vi "读取检测值.vi"(8 "error in (no error)":errorcluster caption="错误输入（无错误）", 11 "DGUS输入":refnum<class "DGUS.lvclass">) -> (0 "error out":errorcluster caption="错误输出", 2 "检测值":sgl, 3 "DGUS输出":refnum<class "DGUS.lvclass">)   [LabVIEW 2016, in "DGUS.lvlib" / "DGUS.lvclass"]
uses:
  DGUS.lvclass
  DGUS.lvclass/DGUS.ctl
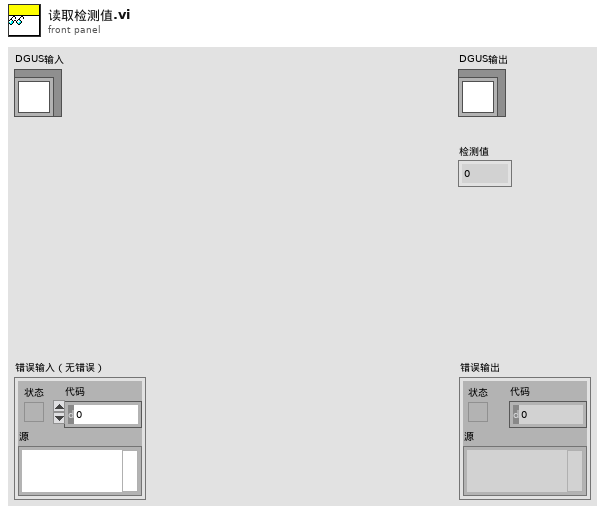
[diagram p1: front panel]
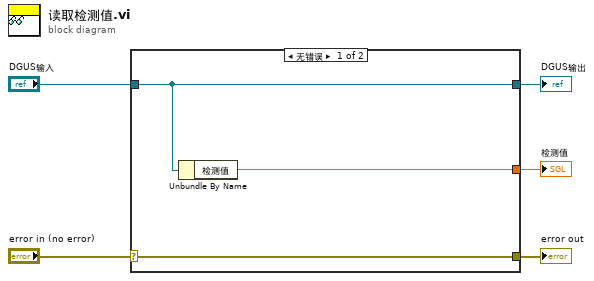
[diagram p0: block diagram]
diagram:
  n1 = case shown="无错误" "error in (no error)" {
    selector: "error in (no error)" -> [w8 w9]
    tunnel: [w8 w9] -> w4
    tunnel: [w7 w10] -> w2
    tunnel: "DGUS输入" -> [w7 w10]
    tunnel: [w6 _] -> w1
    frame No Error {
      n2 = Unbundle By Name(w7) -> ("检测值"=w6:sgl)
    }
    frame Error {
    }
  }
  "error out" <- w4
  "DGUS输出" <- w2
  "检测值" <- w1
